vi "R_Index_search.vi"(5 "Regex":string, 11 "error in (no error)":errorcluster) -> (3 "match":string[](array[string]), 4 "before match":string[](array[string]), 6 "keys":string[](array[string]), 8 "after match":string[](array[string]), 10 "Match ?":bool, 13 "How many":i32, 14 "Match index":i32[](array[numeric]), 15 "error out":errorcluster)   [LabVIEW 2015]
uses:
  <vilib>/regexp/Match Regular Expression.xnode
panel:
  out "Key_index":string[](array[string])
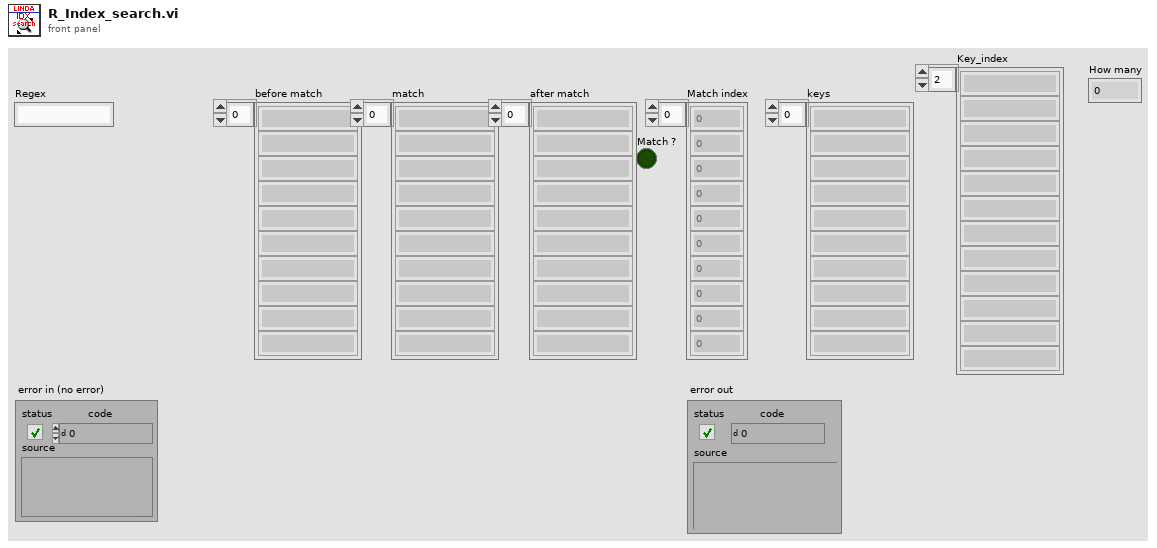
[diagram p1: front panel]
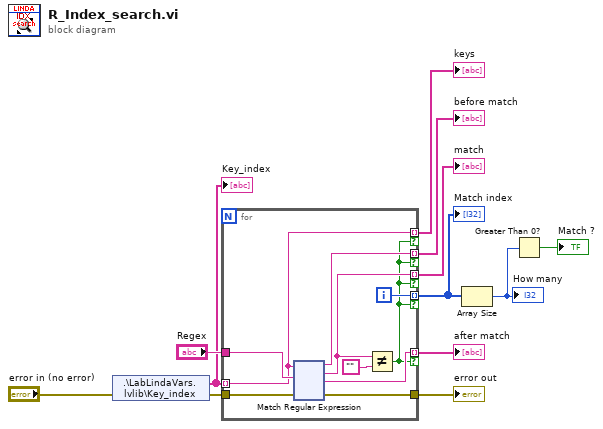
[diagram p0: block diagram]
diagram:
  n1 = shared-variable ".\\LabLindaVars.lvlib\\Key_index"(error in="error in (no error)") -> (w8:string[], error out=w1:errorcluster)
  "Key_index" <- w8
  n2 = for {
    tunnel: w8 -> [w15] mode=indexing
    tunnel: "Regex" -> [w22]
    tunnel: [w21] -> w9 mode=indexing if=w16
    tunnel: [w19] -> w10 mode=indexing if=w16
    tunnel: [w20] -> w11 mode=indexing if=w16
    tunnel: [w17] -> w7 mode=indexing if=w16
    tunnel: [w15] -> w3 mode=indexing if=w16
    tunnel: w1 -> [w14]
    tunnel: [w13] -> w4
    i -> [w17]
    n3 = xnode "Match Regular Expression"("input string"=w15, "regular expression"=w22, "error in"=w14) -> ("before match"=w20:string, "whole match"=w19:string, "after match"=w21:string, "error out"=w13:errorcluster)  [unwired: 3 in, 1 out]
    n4 = Not Equal?(x=w19, y="") -> (x != y?=w16:bool)
  }
  "before match" <- w11
  "match" <- w10
  "after match" <- w9
  "Match index" <- w7
  "error out" <- w4
  "keys" <- w3
  n5 = Array Size(array=w7) -> (size(s)=w6:i32)
  "How many" <- w6
  n6 = Greater Than 0?(x=w6) -> (x > 0?=→"Match ?":bool)
